vi "VI Broken.vi"(8 "error in (no error)":errorcluster, 11 "vi ref in":refnum<vi>) -> (0 "error out":errorcluster, 2 "broken?":bool, 3 "vi ref out":refnum<vi>)   [LabVIEW 2020, in "Build Automation.lvlib"]
uses:
  Build Automation.lvlib
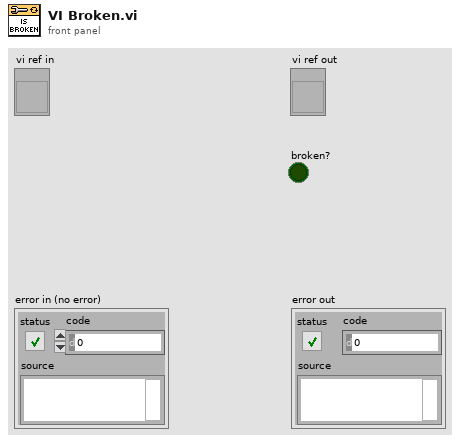
[diagram p1: front panel]
types:
  T1 = enum32{"Bad", "Idle", "Run top level", "Running"}
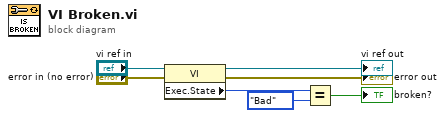
[diagram p0: block diagram]
diagram:
  n1 = property class="VI"(reference="vi ref in", error in="error in (no error)") -> (reference out=→"vi ref out":refnum<vi>, error out=→"error out":errorcluster, "Exec.State"=w3:T1)
  n2 = Equal?(x=w3, y=T1."Bad") -> (x = y?=→"broken?":bool)
